vi "PH_SRDG645.Close.vi"(0 "i ref in":refnum<vi>, 5 "error in":errorcluster) -> (14 "i ref out":refnum<vi>, 19 "error out":errorcluster)   [LabVIEW 2014, in "PH_SRDG645.lvlib"]
doc: "This VI closes the connection to the hardware."
uses:
  PH_SRDG645.lvlib
  instr.lib/Stanford Research DG645/Stanford Research DG645 - Driver.lvlib
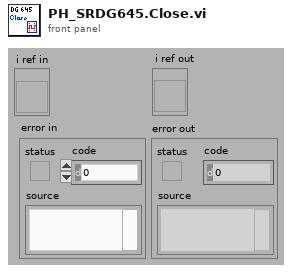
[diagram p1: front panel]
types:
  T1 = typedef "PH_SRDG645.lvlib/PH_SRDG645.i attribute.ctl" = cluster{"GUI Refs":cluster{"Delete":refnum<vi>, "Device Errors":refnum<vi>, "Trigger":refnum<vi>, "Default Name":refnum<vi>, "Firmware Revision":refnum<vi>, "Serial Number":refnum<vi>, "Model":refnum<vi>, "Visa resource name":refnum<vi>}, "Service ID Rate":i32, "Service IDs Channelinfo":i32[], "VISA resource name":refnum<visa-resource-name>, "Device Errors":cluster{"code":i32, "Text":string}[], "Trigger":T2, "Channels":cluster{"T1":T3, "A":T3, "B":T3, "C":T3, "D":T3, "E":T3, "F":T3, "G":T3, "H":T3}, "GUI Refs Channels":refnum<vi>[], "Outputs":cluster{"AB":cluster{"Level Offset [V]":dbl, "Amplitue [V]":dbl, "Polarity":i32}, "CD":cluster{"Level Offset [V]":dbl, "Amplitue [V]":dbl, "Polarity":i32}, "EF":cluster{"Level Offset [V]":dbl, "Amplitue [V]":dbl, "Polarity":i32}, "GH":cluster{"Level Offset [V]":dbl, "Amplitue [V]":dbl, "Polarity":i32}, "T0":cluster{"Level Offset [V]":dbl, "Amplitue [V]":dbl, "Polarity":i32}}, "GUI Refs Outputs":refnum<vi>[], "Serial Number":string, "Firmweare Revision":string, "Model":string}
  T2 = typedef "PH_SRDG645.lvlib/PH_SRDG645.Trigger.ctl" = cluster{"Source":i32, "Rate [Hz]":dbl, "Level [V]":dbl}
  T3 = typedef "PH_SRDG645.lvlib/PH_SRDG645.Channel Settings.ctl" = cluster{"Delay [s]":dbl, "relative to":i32}
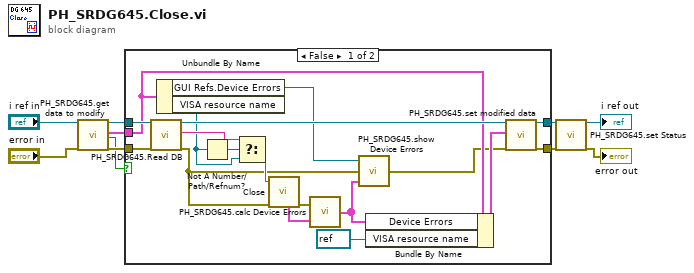
[diagram p0: block diagram]
diagram:
  n1 = call "PH_SRDG645.get data to modify.vi"("i ref in"="i ref in", "error in (no error)"="error in") -> ("i ref out"=w9:refnum<vi>, "i attribute"=w5:T1, "timed out"=w6:bool, "error out"=w7:errorcluster)  [unwired: 14 in]
  n2 = case shown="False" w6 {
    tunnel: w9 -> [w28 w30]
    tunnel: [w27 w29] -> w2
    tunnel: w7 -> [w26 w29]
    tunnel: [w24 w30] -> w4
    tunnel: w5 -> [w22 _]
    frame False {
      n3 = call "PH_SRDG645.Read DB.vi"("i ref in"=w28, "error in"=w26) -> ("i ref out"=w25:refnum<vi>, "Default Name"=w20:string, "error out"=w16:errorcluster)  [unwired: 15 in]
      n4 = Unbundle By Name(w22) -> ("GUI Refs.Device Errors"=w14:refnum<vi>, "VISA resource name"=w19:refnum<visa-resource-name>)
      n5 = Not A Number/Path/Refnum?(number/path/refnum=w19) -> (NaN/Path/Refnum?=w21:bool)
      n6 = Select(t=w20, s=w21, f=w19) -> (s? t:f=w18:string)
      n7 = call "Close.vi"("error in (no error)"=w16, "VISA resource name"=w18) -> ("error out"=w13:errorcluster, "Device Errors"=w12:cluster{"code":i32, "Text":string}[])  [unwired: 8 in]
      n8 = call "PH_SRDG645.calc Device Errors.vi"("Device Errors out"=w12, "SRDG 645 error out"=w13) -> ("calculate Device Errors"=w11:cluster{"code":i32, "Text":string}[])
      n9 = call "PH_SRDG645.show Device Errors.vi"("Device Errors"=w11, "error in"=w16, "Ref Device Errors"=w14) -> ("error out"=w15:errorcluster)
      n10 = Bundle By Name(cluster=w22, "Device Errors"=w11, "VISA resource name"=refnum<visa-resource-name> refnum) -> (w23:T1)
      n11 = call "PH_SRDG645.set modified data.vi"("i ref in"=w25, "i attribute"=w23, "error in (no error)"=w15) -> ("i ref out"=w24:refnum<vi>, "error out"=w27:errorcluster)  [unwired: 15 in]
    }
    frame True {
    }
  }
  n12 = call "PH_SRDG645.set Status.vi"("i ref in"=w4, "error in"=w2) -> ("i ref out"=→"i ref out":refnum<vi>, "error out"=→"error out":errorcluster)  [unwired: 16 in]
